vi "Validate Configuration Metadata.vi"(8 "error in (no error)":errorcluster) -> (0 "error out":errorcluster, 2 "Invalid Parameters":string, 3 "Is Metadata Valid":bool)   [LabVIEW 2020, in "MeasurementLink Measurement Server.lvlib"]
uses:
  MeasurementLink Measurement Server.lvlib
  <vilib>/Utility/Data Type/NI_Data Type.lvlib
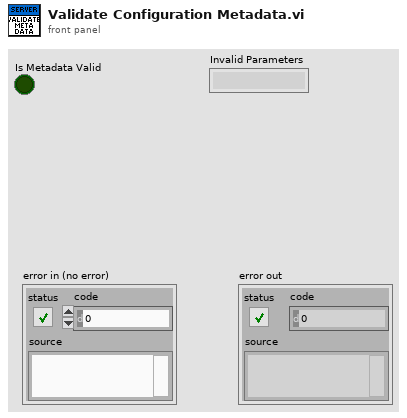
[diagram p1: front panel]
types:
  T1 = typedef "MeasurementLink Measurement Template.lvlib/Measurement Configuration.ctl" = cluster{"Array in":dbl[]}
  T2 = typedef "MeasurementLink Measurement Server.lvlib/Parameter Type Specialization.ctl" = cluster{"Parameter Name":string, "Type Specialization":T3, "Annotations":cluster{"Key":T4, "Value":string}[]}
  T3 = typedef "MeasurementLink Measurement Server.lvlib/Type Specialization.ctl" = enum16{"none", "pin"}
  T4 = typedef "MeasurementLink Measurement Server.lvlib/Key.ctl" = enum16{"none", "pin.instrument_type"}
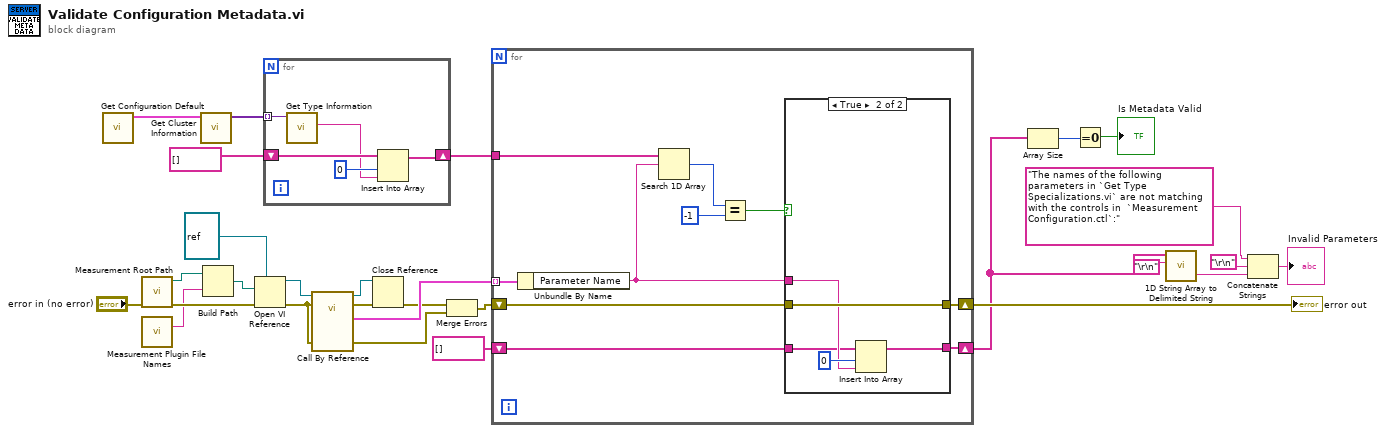
[diagram p0: block diagram]
diagram:
  n1 = call "Get Configuration Default.vi"() -> ("Measurement Configuration Default"=w1:T1)  [unwired: 10 in, 1 out]
  n2 = call "Measurement Root Path.vi"("error in (no error)"="error in (no error)") -> ("error out"=w13:errorcluster, "Measurement Library Path out"=w12:path)  [unwired: 9 in]
  n3 = call "Measurement Plugin File Names.vi"() -> ("Get Type Specializations"=w10:string)  [unwired: 13 in, 2 out]
  n4 = call <vilib>:"Get Cluster Information.vi"("variant"=w1) -> ("cluster elements"=w28:variant[])  [unwired: 9 in, 1 out]
  n5 = Build Path(base path=w12, name or relative path=w10) -> (appended path=w11:path)
  n6 = Open VI Reference(type specifier VI Refnum (for type only)=refnum<vi> refnum, vi path=w11, error in (no error)=w13) -> (vi reference=w15:refnum<vi>, error out=w7:errorcluster)  [unwired: 3 in]
  n7 = for {
    tunnel: w28 -> [w33] mode=indexing
    shift-right: [w29] -> w26
    shift-left: string[] [] -> [w31]
    n8 = call <vilib>:"Get Type Information.vi"("variant"=w33) -> ("name"=w30:string)  [unwired: 6 in, 4 out]
    n9 = Insert Into Array(array=w31, index=0, new element=w30) -> (w29:string[])
  }
  n10 = call-by-ref "?"(reference=w15, error in=w7, 8:"error in (no error)"=w7) -> (reference out=w8:refnum<vi>, error out=w9:errorcluster, 0:"error out"=w2:errorcluster, "Type Specializations"=w6:T2[])  [unwired: 9 in]
  n11 = Close Reference(reference=w8, error in (no error)=w9) -> (error out=w3:errorcluster)
  n12 = Merge Errors(w3, w2) -> (w4:errorcluster)
  n13 = for {
    tunnel: w6 -> [w43] mode=indexing
    shift-right: [w37] -> w24
    shift-left: w4 -> [w38]
    tunnel: w26 -> [w42]
    shift-right: [w34] -> w17
    shift-left: string[] [] -> [w36]
    n14 = Unbundle By Name(w43) -> ("Parameter Name"=w35:string)
    n15 = Search 1D Array(1D array=w42, element=w35) -> (index of element=w41:i32)  [unwired: 1 in]
    n16 = Equal?(x=w41, y=-1) -> (x = y?=w39:bool)
    n17 = case shown="True" w39 {
      tunnel: w38 -> [w45 w50]
      tunnel: [w45 w50] -> w37
      tunnel: w36 -> [w44 w47]
      tunnel: w35 -> [_ w48]
      tunnel: [w44 w46] -> w34
      frame False {
      }
      frame True {
        n18 = Insert Into Array(array=w47, index=0, new element=w48) -> (w46:string[])
      }
    }
  }
  "error out" <- w24
  n19 = Array Size(array=w17) -> (size(s)=w23:i32)
  n20 = Equal To 0?(x=w23) -> (x = 0?=→"Is Metadata Valid":bool)
  n21 = call <vilib>:"1D String Array to Delimited String.vi"("delimiter"="\r\n", "string array"=w17) -> ("delimited string"=w18:string)  [unwired: 9 in]
  n22 = Concatenate Strings("The names of the following parameters in `Get Type Specializations.vi` are not matching with the controls in  `Measurement Configuration.ctl`:" ("string"), "\r\n", w18) -> (→"Invalid Parameters":string)
